vi "Main.vi"() -> ()   [LabVIEW 2014]
uses:
  Controls/State Variables.ctl
  Controls/DAQmx Variables.ctl
  Controls/Filter Variables.ctl
  <vilib>/DAQmx/read.llb/DAQmx Read (Analog 2D DBL NChan NSamp).vi
  <vilib>/DAQmx/miscellaneous.llb/DAQmx Fill In Error Info.vi
  <vilib>/addons/Wavelet Analysis/application.llb/WA Denoise (DWT Real Array).vi
  <vilib>/measure/mamon.llb/Trigger Detection for 1 Channel.vi
  Support VIs/ECG Input.lvlib
  Support VIs/Filter.lvlib
  <vilib>/addons/_Advanced Signal Processing/NI_AdvSigProcWA.lvlib
  Support VIs/Flow Control.lvlib
  <vilib>/measure/NI_MAPro.lvlib
  Support VIs/Trigger Output.lvlib
panel:
  in  "Trigger Delay":u16 caption="Delay" max=500 step=1 format="%#.0p ms"
  in  "Triggers per Shot":i32(knob)=1 caption="shots" scale=1.0..5.0
  out "Start Trigger":bool
  out "Test View":dbl[](graph)
  in  "Reset Button":bool
  in  "Trigger Output":tag
  in  "ECG Input":tag
  in  "Trigger Level":dbl(slide) scale=0.0..1.0
  in  "Exit Button":bool
  in  "Arm Button":bool
  in  "Set Button":bool
  out "Signal Viewer":dbl[][](graph)
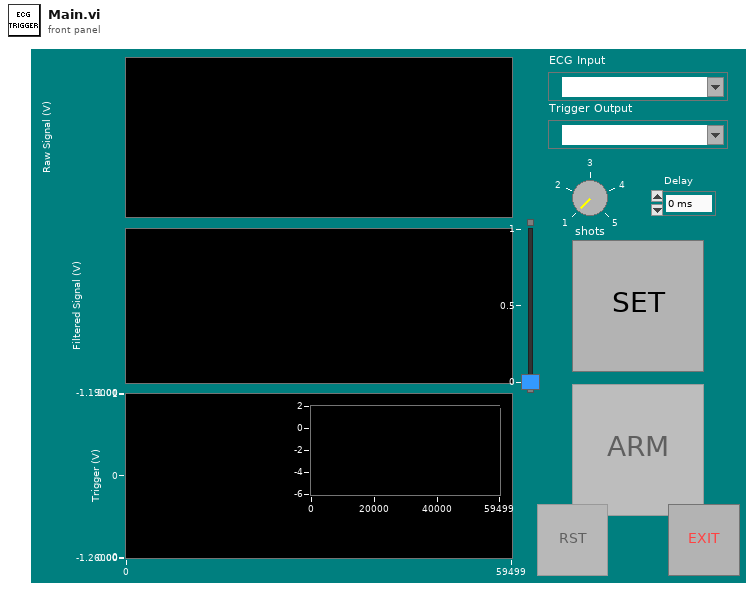
[diagram p1: front panel]
types:
  T1 = typedef "State Variables.ctl" = cluster{"Stop Notifier":refnum<notifier>, "UI References":refnum<vi>[], "DAQmx":T2, "Data Queue":refnum<queue>, "Filter":T3, "Last Detect Result":bool}
  T2 = typedef "DAQmx Variables.ctl" = cluster{"ECG Input":cluster{"Channel":tag, "Task":refnum<k21>, "Max Value":dbl, "Min Value":dbl, "Sampling Rate":dbl, "Batch Size":i32}, "Trigger Output":cluster{"Channel":tag, "Task":refnum<k21>, "Pulse Frequency":dbl, "Delay":u16, "Triggers per Shot":i32}}
  T3 = typedef "Filter Variables.ctl" = cluster{"Batch Size":i32, "Update Cycle":i32, "Filter Buffer":dbl[]}
  T4 = typedef "LVRangeTypeDef.ctl" = cluster{"Minimum":dbl, "Maximum":dbl, "Increment":dbl, "Minor Increment":dbl, "Start":dbl}
  T5 = cluster{"thresholding rule":enum16{"SURE", "Hybrid", "Universal", "Minimax"}, "rescaling method":u16, "soft threshold?":bool}
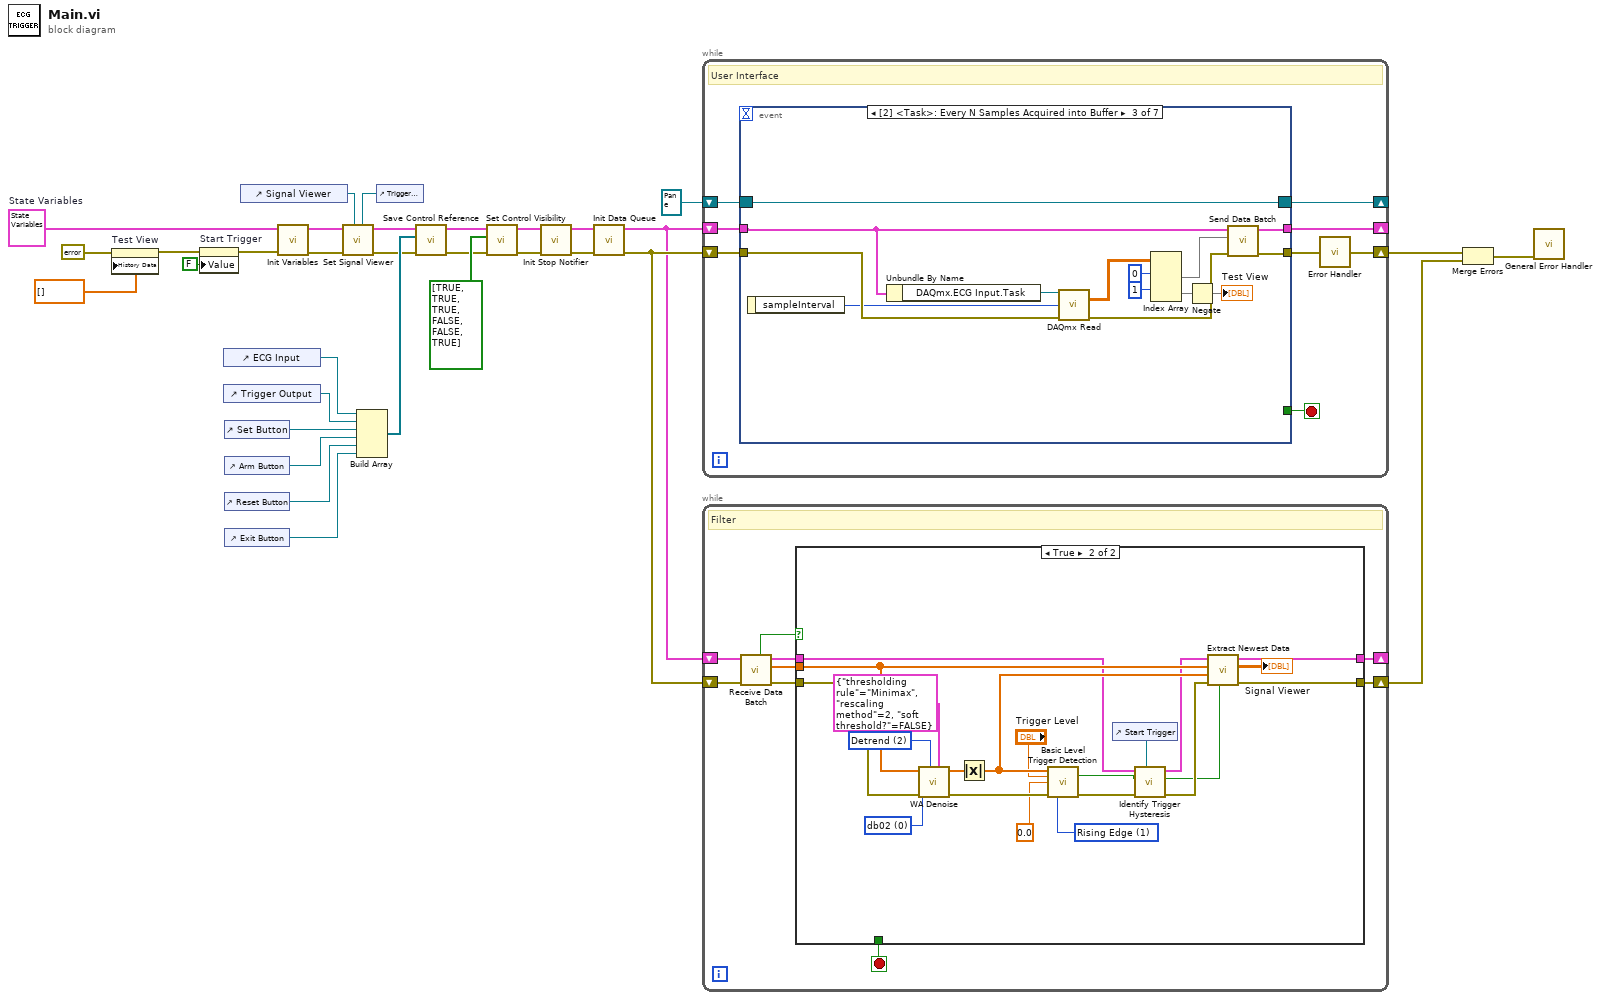
[diagram p0: block diagram]
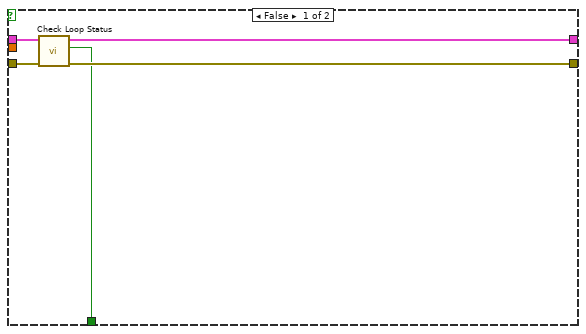
[diagram p2: hidden frame]
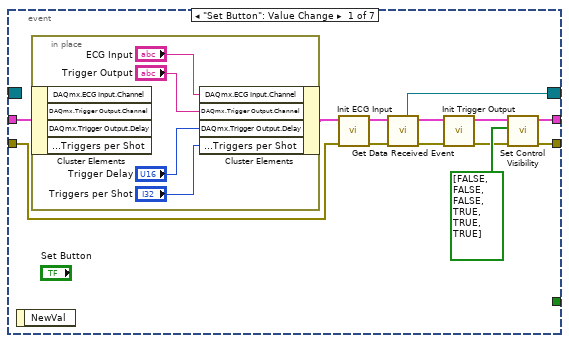
[diagram p3: hidden frame]
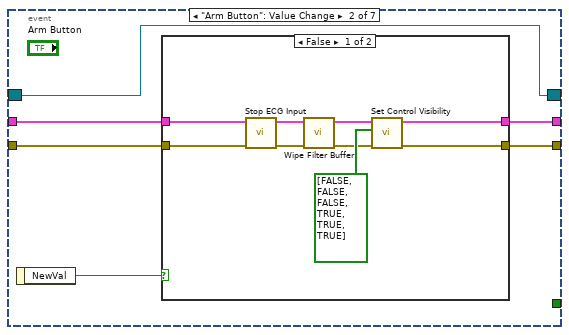
[diagram p4: hidden frame]
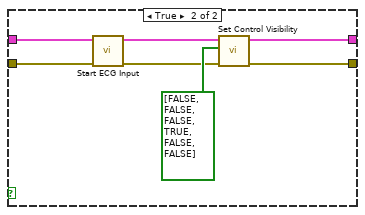
[diagram p5: hidden frame]
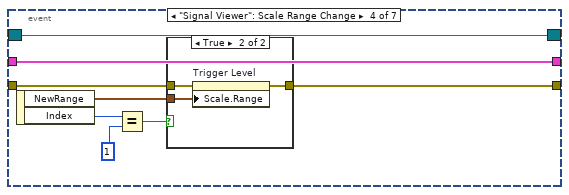
[diagram p6: hidden frame]
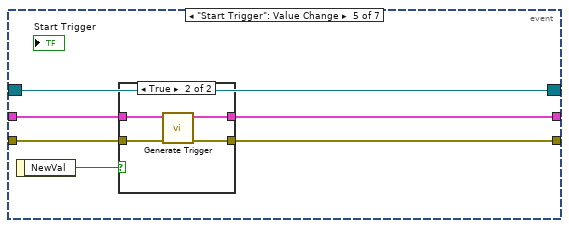
[diagram p8: hidden frame]
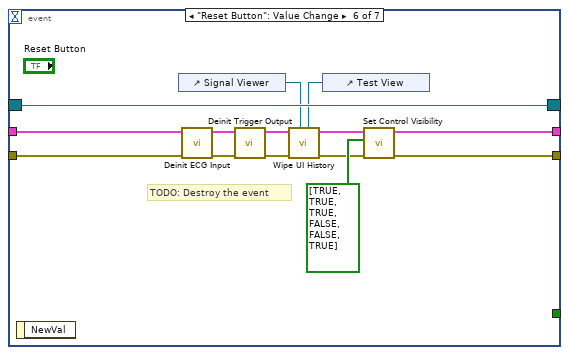
[diagram p10: hidden frame]
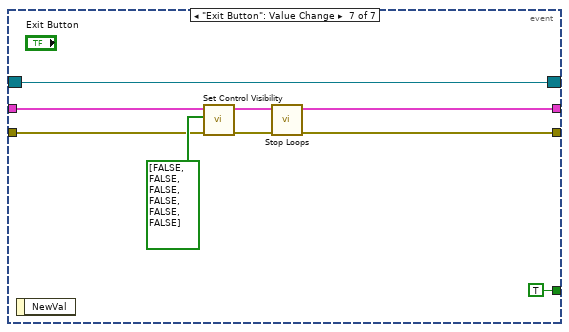
[diagram p11: hidden frame]
diagram:
  w16 = T1 {"Stop Notifier"=refnum, "UI References"=[], "DAQmx"={"ECG Input"={"Channel"="", "Task"="", "Max Value"=0.0, "Min Value"=0.0, "Sampling Rate"=0.0, "Batch Size"=0}, "Trigger Output"={"Channel"="", "Task"="", "Pulse Frequency"=0.0, "Delay"=0, "Triggers per Shot"=0}}, "Data Queue"=refnum, "Filter"={"Batch Size"=0, "Update Cycle"=0, "Filter Buffer"=[]}, "Last Detect Result"=FALSE}  # State Variables
  n1 = property on="Test View" class="WFChart (strict)"(error in=errorcluster {"status"=FALSE, "code"=0, "source"=""} ("error constant"), "History Data"=dbl[] []) -> (error out=w4:errorcluster)  [unwired: 1 in, 1 out]
  n2 = property on="Start Trigger" class="Bool (strict)"(error in=w4, "Value"=FALSE ("Start Trigger")) -> (error out=w5:errorcluster)  [unwired: 1 in, 1 out]
  n3 = control-ref of="ECG Input"() -> (w31:refnum<vi>)
  n4 = control-ref of="Trigger Output"() -> (w30:refnum<vi>)
  n5 = control-ref of="Set Button"() -> (w29:refnum<vi>)
  n6 = control-ref of="Arm Button"() -> (w28:refnum<vi>)
  n7 = control-ref of="Reset Button"() -> (w27:refnum<vi>)
  n8 = control-ref of="Exit Button"() -> (w26:refnum<vi>)
  n9 = control-ref of="Signal Viewer"() -> (w7:refnum<vi>)
  n10 = call "Init Variables.vi"("Error in"=w5, "State Variables in"=w16) -> ("Error out"=w8:errorcluster, "State Variables out"=w11:T1)  [unwired: 8 in]
  n11 = Build Array(w31, w30, w29, w28, w27, w26) -> (w32:refnum<vi>[])
  n12 = control-ref of="Trigger Level"() -> (w6:refnum<vi>)
  n13 = call "Set Signal Viewer.vi"("Trigger Level Reference"=w6, "Signal Viewer Reference"=w7, "Error in"=w8, "State Variables in"=w11) -> ("Error out"=w9:errorcluster, "State Variables out"=w10:T1)  [unwired: 6 in]
  n14 = call "Save Control Reference.vi"("Error in"=w9, "Reference Input"=w32, "State Variables in"=w10) -> ("Error out"=w19:errorcluster, "State Variables out"=w20:T1)  [unwired: 7 in]
  n15 = call "Set Control Visibility.vi"("Error in"=w19, "States of Controls"=bool[] [TRUE, TRUE, TRUE, FALSE, FALSE, TRUE], "State Variables in"=w20) -> ("Error out"=w22:errorcluster, "State Variables out"=w21:T1)  [unwired: 7 in]
  n16 = call "Init Stop Notifier.vi"("Error in"=w22, "State Variables in"=w21) -> ("Error out"=w24:errorcluster, "State Variables out"=w25:T1)  [unwired: 8 in]
  n17 = call "Init Data Queue.vi"("Error in"=w24, "State Variables in"=w25) -> ("Error out"=w2:errorcluster, "State Variables out"=w1:T1)  [unwired: 8 in]
  n18 = while {
    shift-right: [w39] -> _
    shift-left: w1 -> [w40]
    shift-right: [w34] -> w18
    shift-left: w2 -> [w38]
    shift-right: [w37] -> _
    shift-left: refnum<event-registration> refnum ("RegEvent Refnum") -> [w36]
    stop <- w33 stop-if-true
    # "User Interface"
    n19 = event shown="[2] <Task>: Every N Samples Acquired into Buffer" {
      selector: w36 -> [_ w58 w86 w95 w111 w128 w133]
      dyn-events: [w45 w58 w86 w95 w111 w128 w133] -> w37
      timeout: _ -> [_ _ _ _ _ _ _]
      tunnel: w40 -> [w48 w62 w89 w96 w110 w127 w139]
      tunnel: [w53 w60 w90 w96 w107 w129 w134] -> w39
      tunnel: w38 -> [w46 w61 w88 w100 w109 w126 w138]
      tunnel: [w52 w59 w91 w99 w108 w130 w135] -> w35
      tunnel: [_ _ _ _ _ _ TRUE] -> w33
      event "Set Button": Value Change {
        n20 = event-data() -> ()  [unwired: 1 in, 1 out]
        n21 = in-place {
          n22 = in-place-cluster #1(w48) -> ()  [unwired: 4 out]
          n23 = in-place-cluster #1("DAQmx.ECG Input.Channel"="ECG Input", "DAQmx.Trigger Output.Channel"="Trigger Output", "DAQmx.Trigger Output.Delay"="Trigger Delay", "DAQmx.Trigger Output.Triggers per Shot"="Triggers per Shot") -> (w47:T1)
        }
        n24 = call "Init ECG Input.vi"("Error in"=w46, "State Variables in"=w47) -> ("Error out"=w49:errorcluster, "State Variables out"=w50:T1)  [unwired: 8 in]
        n25 = call "Get Data Received Event.vi"("Error in"=w49, "State Variables in"=w50) -> ("Error out"=w43:errorcluster, "State Variables out"=w44:T1, "RegEvent Refnum"=w45:refnum<event-registration>)  [unwired: 7 in]
        n26 = call "Init Trigger Output.vi"("Error in"=w43, "State Variables in"=w44) -> ("Error out"=w42:errorcluster, "State Variables out"=w41:T1)  [unwired: 8 in]
        n27 = call "Set Control Visibility.vi"("Error in"=w42, "States of Controls"=bool[] [FALSE, FALSE, FALSE, TRUE, TRUE, TRUE], "State Variables in"=w41) -> ("Error out"=w52:errorcluster, "State Variables out"=w53:T1)  [unwired: 7 in]
      }
      event "Arm Button": Value Change {
        n28 = event-data() -> ("NewVal"=w63:bool)  [unwired: 1 in]
        n29 = case shown="False" w63 {
          tunnel: w62 -> [w69 w76]
          tunnel: w61 -> [w68 w75]
          tunnel: [w71 w78] -> w60
          tunnel: [w70 w77] -> w59
          frame False {
            n30 = call "Stop ECG Input.vi"("error in (no error)"=w68, "State Variables in"=w69) -> ("error out"=w67:errorcluster, "State Variables out"=w66:T1)  [unwired: 8 in]
            n31 = call "Wipe Filter Buffer.vi"("Error in"=w67, "State Variables in"=w66) -> ("Error out"=w64:errorcluster, "State Variables out"=w65:T1)  [unwired: 8 in]
            n32 = call "Set Control Visibility.vi"("Error in"=w64, "States of Controls"=bool[] [FALSE, FALSE, FALSE, TRUE, TRUE, TRUE], "State Variables in"=w65) -> ("Error out"=w70:errorcluster, "State Variables out"=w71:T1)  [unwired: 7 in]
          }
          frame True {
            n33 = call "Start ECG Input.vi"("error in (no error)"=w75, "State Variables in"=w76) -> ("error out"=w73:errorcluster, "State Variables out"=w74:T1)  [unwired: 8 in]
            n34 = call "Set Control Visibility.vi"("Error in"=w73, "States of Controls"=bool[] [FALSE, FALSE, FALSE, TRUE, FALSE, FALSE], "State Variables in"=w74) -> ("Error out"=w77:errorcluster, "State Variables out"=w78:T1)  [unwired: 7 in]
          }
        }
      }
      event Every N Samples Acquired into Buffer {
        n35 = event-data() -> ("sampleInterval"=w87:u32)  [unwired: 1 in]
        n36 = Unbundle By Name(w89) -> ("DAQmx.ECG Input.Task"=w93:refnum<k21>)
        n37 = call-poly <vilib>:"DAQmx Read.vi"("task/channels in"=w93, "number of samples per channel"=w87, "error in"=w88) -> ("data"=w85:dbl[][], "error out"=w92:errorcluster)  [unwired: 10 in, 1 out]
        n38 = Index Array(array=w85, index (row) #1=0 ("index"), index (row) #2=1 ("index (row)")) -> (element #1=w83:dbl[], element #2=w81:dbl[])  [unwired: 2 in]
        n39 = Negate(x=w81) -> (-x=→"Test View":dbl[])
        n40 = call "Send Data Batch.vi"("Error in"=w92, "New Data"=w83, "State Variables in"=w89) -> ("Error out"=w91:errorcluster, "State Variables out"=w90:T1)  [unwired: 7 in]
      }
      event "Signal Viewer": Scale Range Change {
        n41 = event-data() -> ("NewRange"=w101:T4, "Index"=w98:i32)  [unwired: 1 in]
        n42 = Equal?(x=w98, y=1) -> (x = y?=w94:bool)
        n43 = case shown="True" w94 {
          tunnel: w101 -> [_ w105]
          tunnel: w100 -> [w102 w104]
          tunnel: [w102 w103] -> w99
          frame False {
          }
          frame True {
            n44 = property on="Trigger Level" class="Slide (strict)"(error in=w104, "Scale.Range"=w105) -> (error out=w103:errorcluster)  [unwired: 1 in, 1 out]
          }
        }
      }
      event "Start Trigger": Value Change {
        n45 = event-data() -> ("NewVal"=w106:bool)  [unwired: 1 in]
        n46 = case shown="True" w106 {
          tunnel: w110 -> [w113 w117]
          tunnel: w109 -> [w112 w116]
          tunnel: [w112 w115] -> w108
          tunnel: [w113 w114] -> w107
          frame False {
          }
          frame True {
            n47 = call "Generate Trigger.vi"("Error in"=w116, "State Variables in"=w117) -> ("Error out"=w115:errorcluster, "State Variables out"=w114:T1)  [unwired: 8 in]
          }
        }
      }
      event "Reset Button": Value Change {
        # "TODO: Destroy the event"
        n48 = event-data() -> ()  [unwired: 1 in, 1 out]
        n49 = control-ref of="Signal Viewer"() -> (w119:refnum<vi>)
        n50 = call "Deinit ECG Input.vi"("Error in"=w126, "State Variables in"=w127) -> ("Error out"=w124:errorcluster, "State Variables out"=w123:T1)  [unwired: 8 in]
        n51 = call "Deinit Trigger Output.vi"("Error in"=w124, "State Variables in"=w123) -> ("Error out"=w122:errorcluster, "State Variables out"=w120:T1)  [unwired: 8 in]
        n52 = control-ref of="Test View"() -> (w118:refnum<vi>)
        n53 = call "Wipe UI History.vi"("Secondary Chart"=w118, "Primary Chart"=w119, "Error in"=w122, "State Variables in"=w120) -> ("error out"=w125:errorcluster, "State Variables out"=w121:T1)  [unwired: 6 in]
        n54 = call "Set Control Visibility.vi"("Error in"=w125, "States of Controls"=bool[] [TRUE, TRUE, TRUE, FALSE, FALSE, TRUE], "State Variables in"=w121) -> ("Error out"=w130:errorcluster, "State Variables out"=w129:T1)  [unwired: 7 in]
      }
      event "Exit Button": Value Change {
        n55 = event-data() -> ()  [unwired: 1 in, 1 out]
        n56 = call "Set Control Visibility.vi"("Error in"=w138, "States of Controls"=bool[] [FALSE, FALSE, FALSE, FALSE, FALSE, FALSE], "State Variables in"=w139) -> ("Error out"=w137:errorcluster, "State Variables out"=w136:T1)  [unwired: 7 in]
        n57 = call "Stop Loops.vi"("Error in"=w137, "State Variables in"=w136) -> ("Error out"=w135:errorcluster, "State Variables out"=w134:T1)  [unwired: 8 in]
      }
    }
    n58 = call "Error Handler.vi"("Error in"=w35) -> ("Error out"=w34:errorcluster)  [unwired: 2 in, 1 out]
  }
  n59 = while {
    shift-right: [w144] -> _
    shift-left: w1 -> [w149]
    shift-right: [w145] -> w14
    shift-left: w2 -> [w148]
    stop <- w142 stop-if-true
    # "Filter"
    n60 = call "Receive Data Batch.vi"("Error in"=w148, "State Variables in"=w149) -> ("Error out"=w146:errorcluster, "Buffered Data"=w141:dbl[], "State Variables out"=w147:T1, "Ready?"=w143:bool)  [unwired: 6 in]
    n61 = case shown="True" w143 {
      tunnel: w147 -> [w153 w161]
      tunnel: w146 -> [w154 w175]
      tunnel: [w151 w170] -> w145
      tunnel: [w152 w171] -> w144
      tunnel: [w150 _] -> w142
      tunnel: w141 -> [_ w165]
      frame False {
        n62 = call "Check Loop Status.vi"("Error in"=w154, "State Variables in"=w153) -> ("Error out"=w151:errorcluster, "Stop Loop?"=w150:bool, "State Variables out"=w152:T1)  [unwired: 7 in]
      }
      frame True {
        w163 = u16 1 items=["Falling Edge", "Rising Edge"] ("trigger slope")
        w172 = u16 0 items=["db02"=0, "db03"=1, "db04"=2, "db05"=3, "db06"=4, "db07"=5, "db08"=6, "db09"=7, "db10"=8, "db11"=9, "db12"=10, "db13"=11, "db14"=12, "Haar"=13, "bior1_3"=14, "bior1_5"=15, "bior2_2"=16, "bior2_4"=17, "bior2_6"=18, "bior2_8"=19, "bior3_1"=20, "bior3_3"=21, "bior3_5"=22, "bior3_7"=23, "bior3_9"=24, "bior4_4 (FBI)"=25, "bior5_5"=38, "bior6_8"=39, "coif1"=26, "coif2"=27, "coif3"=28, "coif4"=29, "coif5"=30, "sym2"=31, "sym3"=32, "sym4"=33, "sym5"=34, "sym6"=35, "sym7"=36, "sym8"=37] ("wavelet")
        w174 = u16 2 items=["None", "Threshold", "Detrend"] ("option for approx coef")
        n63 = call-poly <vilib>:"WA Denoise.vi"("threshold settings"=T5 {"thresholding rule"=enum."Minimax", "rescaling method"=2, "soft threshold?"=FALSE}, "option for approx coef"=w174, "error in (no error)"=w175, "wavelet"=w172, "signal"=w165) -> ("error out"=w167:errorcluster, "denoised signal"=w169:dbl[])  [unwired: 5 in]
        n64 = Absolute Value(x=w169) -> (abs(x)=w166:dbl[])
        n65 = call-poly <vilib>:"Basic Level Trigger Detection.vi"("signal in"=w166, "level"="Trigger Level", "hysteresis"=0.0, "error in (no error)"=w167, "trigger slope"=w163) -> ("trigger detected?"=w160:bool, "error out"=w159:errorcluster)  [unwired: 8 in, 1 out]
        n66 = control-ref of="Start Trigger"() -> (w156:refnum<vi>)
        n67 = call "Identify Trigger Hysteresis.vi"("Start Trigger Refnum"=w156, "Error in"=w159, "Detection Result"=w160, "State Variables in"=w161) -> ("Error out"=w158:errorcluster, "Hysteresis Trigger"=w155:bool, "State Variables out"=w157:T1)  [unwired: 5 in]
        n68 = call "Extract Newest Data.vi"("Triggered?"=w155, "Error in"=w158, "Filtered Signal"=w166, "Raw Signal"=w165, "State Variables in"=w157) -> ("Error out"=w170:errorcluster, "Chart out"=→"Signal Viewer":dbl[][], "State Variables out"=w171:T1)  [unwired: 4 in]
      }
    }
  }
  n69 = Merge Errors(w18, w14) -> (w17:errorcluster)
  n70 = call <vilib>:"General Error Handler.vi"("error in (no error)"=w17) -> ()  [unwired: 10 in, 5 out]
